vi "72_Vision_RC Servo_DC_Moto.vi"() -> ()   [LabVIEW 2018]
uses:
  <userlib>/KNR OS 4.0 LabVIEW Toolkit/Type Definition/Resource.ctl
  <userlib>/KNR OS 4.0 LabVIEW Toolkit/Type Definition/RC Servo Port.ctl
  <userlib>/KNR OS 4.0 LabVIEW Toolkit/Type Definition/DC Motor Port.ctl
panel:
  out "w":dbl
  out "area":dbl
  out "appended array":u16[](array[numeric])
  out "Image Out":T1(plugin-control)
  in  "stop":bool
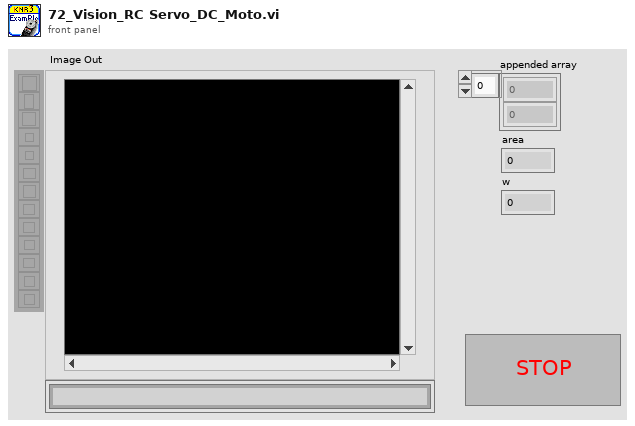
[diagram p1: front panel]
types:
  T1 = typedef "IMAQ Image.ctl" = refnum<image>
  T2 = typedef "RC Servo Port.ctl" = u16
  T3 = typedef "Resource.ctl" = enum16{"KNRm_DDRC", "KNRm_DDDD", "KNRm_DDDR", "KNRm_DDDC", "KNR", "KNRm_neww"}
  T4 = typedef "KNR3 Reference.ctl" = cluster{"FPGA Session":refnum<class "FPGA Interface Base.lvclass">, "Resource":T3}
  T5 = typedef "DC Motor Port.ctl" = u16
  T6 = cluster{"Left":dbl, "Top":dbl, "Right":dbl, "Bottom":dbl}
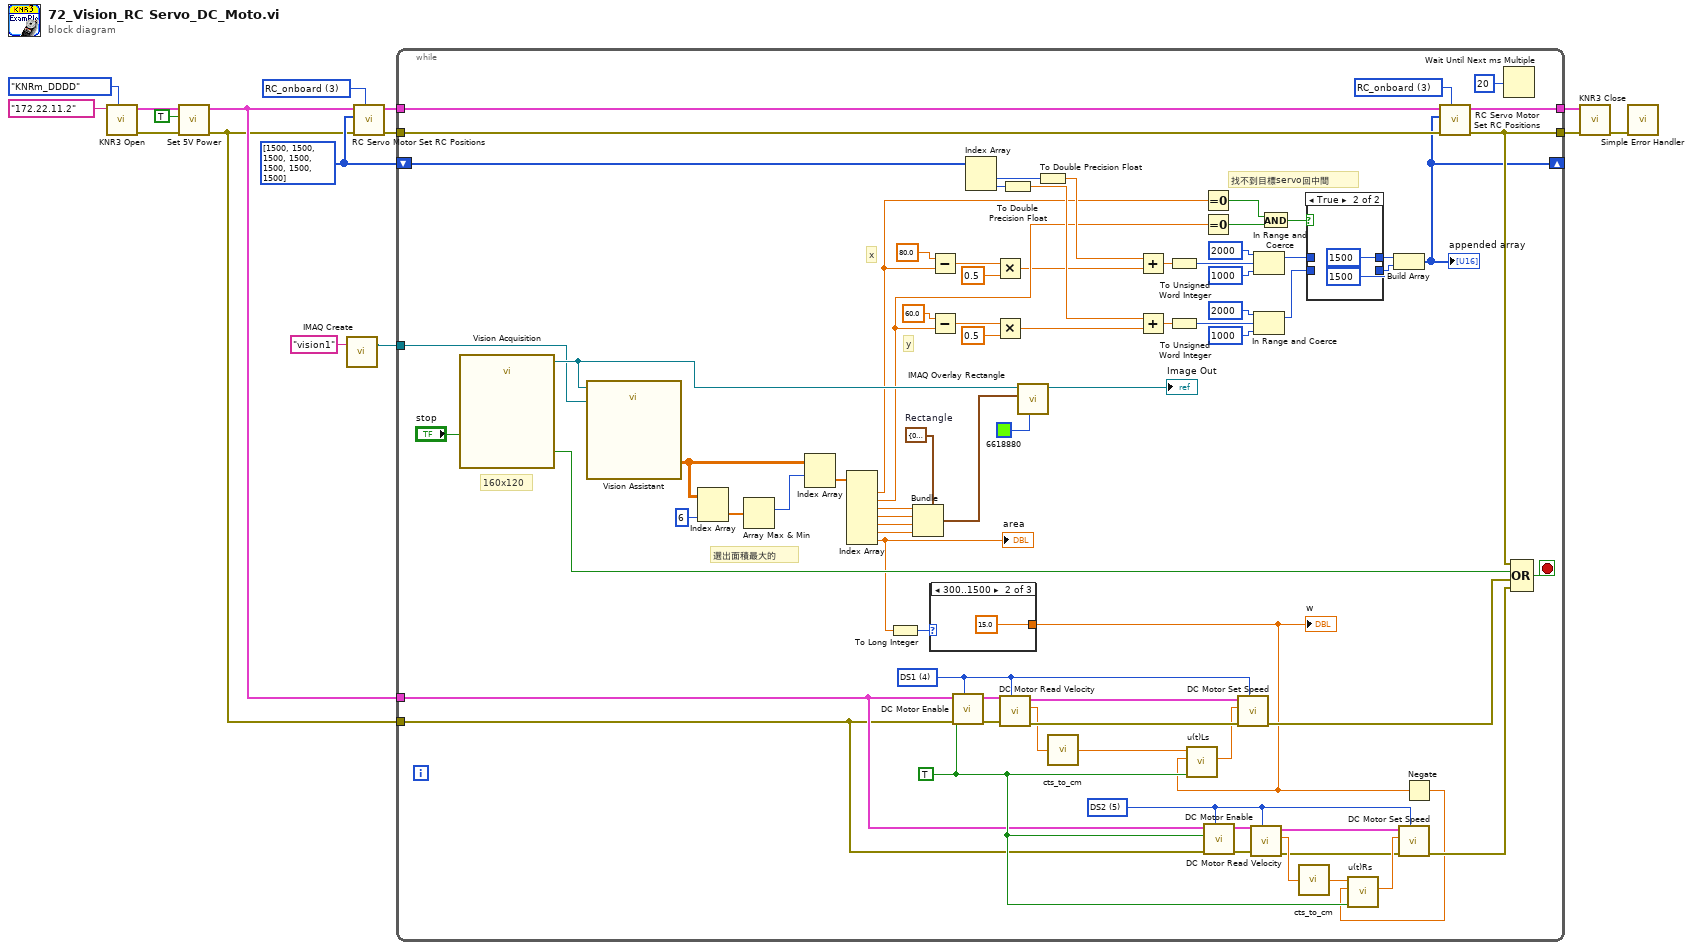
[diagram p0: block diagram]
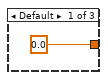
[diagram p2: hidden frame]
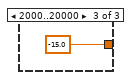
[diagram p3: hidden frame]
diagram:
  w3 = u16[] [1500, 1500, 1500, 1500, 1500, 1500, 1500] ("RC Pulse Width (1500 uS)")
  w6 = T2 3 items=["RC_onboard"=3, "RC_box"=9] ("Port (RC_onboard)")
  n1 = call <userlib>:"KNR3 Open.vi"("Resource"=Resource."KNRm_DDDD", "IP"="172.22.11.2") -> ("error out"=w14:errorcluster, "KNR out"=w15:T4)  [unwired: 8 in]
  n2 = call <userlib>:"Set 5V Power.vi"("error in (no error)"=w14, "5V Power(T)"=TRUE ("5V Power"), "KNR in"=w15) -> ("error out"=w1:errorcluster, "KNR out"=w2:T4)  [unwired: 7 in]
  n3 = call "IMAQ Create"("Image Name"="vision1") -> ("New Image"=w4:T1)  [unwired: 4 in, 1 out]
  n4 = call <userlib>:"RC Servo Motor Set RC Positions.vi"("Port (RC_onboard)"=w6, "RC Pulse Width (1500 uS)"=w3, "KNR in"=w2) -> ("KNR out"=w7:T4)  [unwired: 7 in, 1 out]
  n5 = while {
    tunnel: w7 -> [w95]
    tunnel: [w94] -> w9
    tunnel: w1 -> [w93]
    tunnel: [w91] -> w8
    tunnel: w4 -> [w74]
    shift-right: [w58] -> _
    shift-left: w3 -> [w61]
    tunnel: w2 -> [w20]
    tunnel: w1 -> [w19]
    stop <- w92 stop-if-true
    w24 = T5 5 items=["DS1"=4, "DS2"=5, "DS3"=6, "DS4"=7] ("Port 2")
    w23 = TRUE ("Enable Motor(F)")
    w40 = T5 4 items=["DS1"=4, "DS2"=5, "DS3"=6, "DS4"=7] ("Port 2")
    w87 = T6 {"Left"=0.0, "Top"=0.0, "Right"=0.0, "Bottom"=0.0}  # Rectangle
    w89 = T2 3 items=["RC_onboard"=3, "RC_box"=9] ("RC Motor")
    # "找不到目標servo回中間"
    # "y"
    # "x"
    # "160x120"
    # "選出面積最大的"
    n6 = call "Vision Acquisition"("Stop (F)"="stop") -> ("Image Out"=w79:T1, "Stopped"=w72:bool)  [unwired: 24 in, 1 out]
    n7 = call "Vision Assistant"("Image In"=w79, "Image Dst"=w74) -> ("Particle Measurements (Pixels) (Particle Analysis 1)"=w78:dbl[][])  [unwired: 22 in, 3 out]
    n8 = Index Array "Index Array"(array=w78, index (col)=6 ("disabled index (col)")) -> (element=w77:dbl[])  [unwired: 1 in]
    n9 = Array Max & Min(array=w77) -> (max index (indices)=w76:i32)  [unwired: 3 out]
    n10 = Index Array "Index Array"(array=w78, index (row)=w76) -> (element=w88:dbl[])  [unwired: 1 in]
    n11 = Index Array "Index Array"(array=w88) -> (element #1=w51:dbl, element #2=w50:dbl, element #3=w86:dbl, element #4=w85:dbl, element #5=w84:dbl, element #6=w83:dbl, element #7=w32:dbl)  [unwired: 7 in]
    "area" <- w32
    n12 = To Long Integer(number=w32) -> (32bit integer=w16:i32)
    n13 = Bundle "Bundle"(cluster=w87, "Left"=w86, "Top"=w85, "Right"=w84, "Bottom"=w83) -> (w82:T6)
    n14 = Subtract(x=80.0 ("y"), y=w51) -> (x-y=w68:dbl)
    n15 = Subtract(x=60.0 ("y"), y=w50) -> (x-y=w69:dbl)
    n16 = case shown="300..1500" w16 {
      tunnel: [0.0 15.0 -15.0] -> w17
      frame Default {
      }
      frame 300..1500 {
      }
      frame 2000..20000 {
      }
    }
    "w" <- w17
    n17 = call <userlib>:"DC Motor Enable.vi"("Port (DS1)"=w40, "error in (no error)"=w19, "Enable Motor(F)"=w23, "KNR in"=w20) -> ("error out"=w36:errorcluster, "KNR out"=w35:T4)  [unwired: 6 in]
    n18 = Index Array "Index Array"(array=w61) -> (element #1=w60:u16, element #2=w59:u16)  [unwired: 2 in]
    n19 = Multiply(x=w68, y=0.5) -> (x*y=w49:dbl)
    n20 = Multiply(x=w69, y=0.5) -> (x*y=w48:dbl)
    n21 = call <userlib>:"DC Motor Read Velocity.vi"("Port (DS1)"=w40, "error in (no error)"=w36, "KNR in"=w35) -> ("error out"=w39:errorcluster, "Velocity (cts/sec)"=w37:dbl, "KNR out"=w38:T4)  [unwired: 6 in]
    n22 = To Double Precision Float(number=w59) -> (double precision float=w52:dbl)
    n23 = call "IMAQ Overlay Rectangle"("Color"=u32 6618880, "Rectangle"=w82, "Image"=w79) -> ("Image Out"=→"Image Out":T1)  [unwired: 7 in, 1 out]
    n24 = To Double Precision Float(number=w60) -> (double precision float=w53:dbl)
    n25 = call "cts_to_cm.vi"("cts"=w37) -> ("cm"=w33:dbl)
    n26 = Add(x=w53, y=w49) -> (x+y=w70:dbl)
    n27 = Add(x=w52, y=w48) -> (x+y=w71:dbl)
    n28 = To Unsigned Word Integer(number=w70) -> (unsigned 16bit integer=w55:u16)
    n29 = To Unsigned Word Integer(number=w71) -> (unsigned 16bit integer=w54:u16)
    n30 = call "u(t)Ls.vi"("Velocity"=w33, "Desire Velosity"=w17, "enable"=w23) -> ("u(t)"=w34:dbl)  [unwired: 7 in]
    n31 = Equal To 0?(x=w51) -> (x = 0?=w45:bool)
    n32 = Equal To 0?(x=w50) -> (x = 0?=w46:bool)
    n33 = call <userlib>:"DC Motor Enable.vi"("Port (DS1)"=w24, "error in (no error)"=w19, "Enable Motor(F)"=w23, "KNR in"=w20) -> ("error out"=w28:errorcluster, "KNR out"=w29:T4)  [unwired: 6 in]
    n34 = call <userlib>:"DC Motor Set Speed.vi"("Port (DS1)"=w40, "error in (no error)"=w39, "Speed (+-100%)"=w34, "KNR in"=w38) -> ("error out"=w22:errorcluster)  [unwired: 6 in, 1 out]
    n35 = call <userlib>:"DC Motor Read Velocity.vi"("Port (DS1)"=w24, "error in (no error)"=w28, "KNR in"=w29) -> ("error out"=w25:errorcluster, "Velocity (cts/sec)"=w27:dbl, "KNR out"=w26:T4)  [unwired: 6 in]
    n36 = In Range and Coerce(upper limit=u16 2000, x=w55, lower limit=u16 1000) -> (coerced(x)=w44:u16)  [unwired: 1 out]
    n37 = In Range and Coerce(upper limit=u16 2000, x=w54, lower limit=u16 1000) -> (coerced(x)=w43:u16)  [unwired: 1 out]
    n38 = And(x=w45, y=w46) -> (x .and. y?=w47:bool)
    n39 = call "cts_to_cm.vi"("cts"=w27) -> ("cm"=w31:dbl)
    n40 = case shown="True" w47 {
      tunnel: w44 -> [w100 _]
      tunnel: w43 -> [w99 _]
      tunnel: [w100 u16 1500] -> w42
      tunnel: [w99 u16 1500] -> w41
      frame False {
      }
      frame True {
      }
    }
    n41 = Build Array(w42, w41) -> (w58:u16[])
    "appended array" <- w58
    n42 = Negate(x=w17) -> (-x=w18:dbl)
    n43 = call "u(t)Rs.vi"("Velocity"=w31, "Desire Velosity"=w18, "enable"=w23) -> ("u(t)"=w30:dbl)  [unwired: 7 in]
    n44 = call <userlib>:"DC Motor Set Speed.vi"("Port (DS1)"=w24, "error in (no error)"=w25, "Speed (+-100%)"=w30, "KNR in"=w26) -> ("error out"=w21:errorcluster)  [unwired: 6 in, 1 out]
    n45 = call <userlib>:"RC Servo Motor Set RC Positions.vi"("Port (RC_onboard)"=w89, "error in (no error)"=w93, "RC Pulse Width (1500 uS)"=w58, "KNR in"=w95) -> ("error out"=w91:errorcluster, "KNR out"=w94:T4)  [unwired: 6 in]
    n46 = Wait Until Next ms Multiple(millisecond multiple=u32 20) -> ()  [unwired: 1 out]
    n47 = Compound Arithmetic op=OR(w91, w72, w22, w21) -> (w92:bool)
  }
  n48 = call <userlib>:"KNR3 Close.vi"("error in (no error)"=w8, "KNR in"=w9) -> ("error out"=w13:errorcluster)  [unwired: 9 in]
  n49 = call <vilib>:"Simple Error Handler.vi"("error in (no error)"=w13) -> ()  [unwired: 4 in, 5 out]
